vi "Picolog Run.vi"(8 "Error In":errorcluster, 9 "Interval [s]":dbl=1.0 format="%.2f", 11 "Instrument Handle In":i16=1) -> (0 "Error Out":errorcluster, 1 "Interval [s]":dbl format="%.2f", 3 "Instrument Handle Out":i16)   [LabVIEW 2017]
uses:
  usbtc08.dll
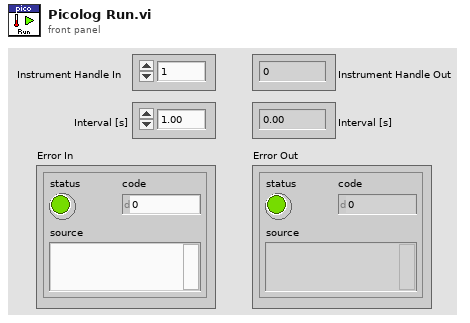
[diagram p1: front panel]
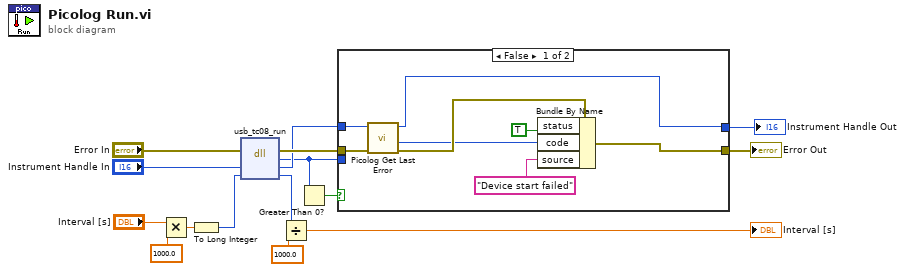
[diagram p0: block diagram]
diagram:
  n1 = Multiply(x="Interval [s]", y=1000.0) -> (x*y=w1:dbl)
  n2 = To Long Integer(number=w1) -> (32bit integer=w2:i32)
  n3 = dll-call lib="usbtc08.dll" fn="usb_tc08_run"(error in="Error In", "handle"="Instrument Handle In", "interval"=w2) -> (error out=w12:errorcluster, "return type"=w5:i32, "handle"=w8:i16, "interval"=w6:i32)  [unwired: 2 in, 1 out]
  n4 = Divide(x=w6, y=1000.0) -> (x/y=→"Interval [s]":dbl)
  n5 = Greater Than 0?(x=w5) -> (x > 0?=w13:bool)
  n6 = case shown="False" w13 {
    tunnel: w5 -> [_ _]
    tunnel: w12 -> [w20 w25]
    tunnel: [w23 w25] -> w11
    tunnel: w8 -> [w18 w24]
    tunnel: [w17 w24] -> w7
    frame False {
      n7 = call "Picolog Get Last Error.vi"("Error In"=w20, "Instrument Handle In"=w18) -> ("Error Out"=w19:errorcluster, "Error Code"=w16:i16, "Instrument Handle Out"=w17:i16)  [unwired: 7 in]
      n8 = Bundle By Name(cluster=w19, "status"=TRUE, "code"=w16, "source"="Device start failed") -> (w23:errorcluster)
    }
    frame True {
    }
  }
  "Error Out" <- w11
  "Instrument Handle Out" <- w7
